vi "Version.vi"(8 "error in (no error)":errorcluster, 11 "S4GUI in":refnum<class "S4GUI.lvclass">) -> (0 "error out":errorcluster, 3 "S4GUI out":refnum<class "S4GUI.lvclass">)   [LabVIEW 2018, in "S4GUI.lvclass"]
uses:
  S4GUI.lvclass
  S4GUI.lvclass/S4GUI.ctl
  SyncBox/Sync Box.lvclass
  Acquisition/Acquisition.lvclass
  Instrument/Instrument.lvclass
  TCS/TCS.lvclass
  TelFocus/TelFocus.lvclass
  WeatherStation/WeatherStation.lvclass
  GSserver/GSserver.lvclass
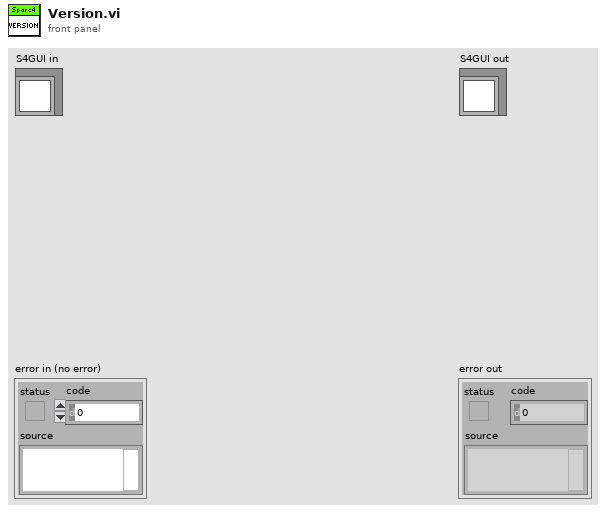
[diagram p1: front panel]
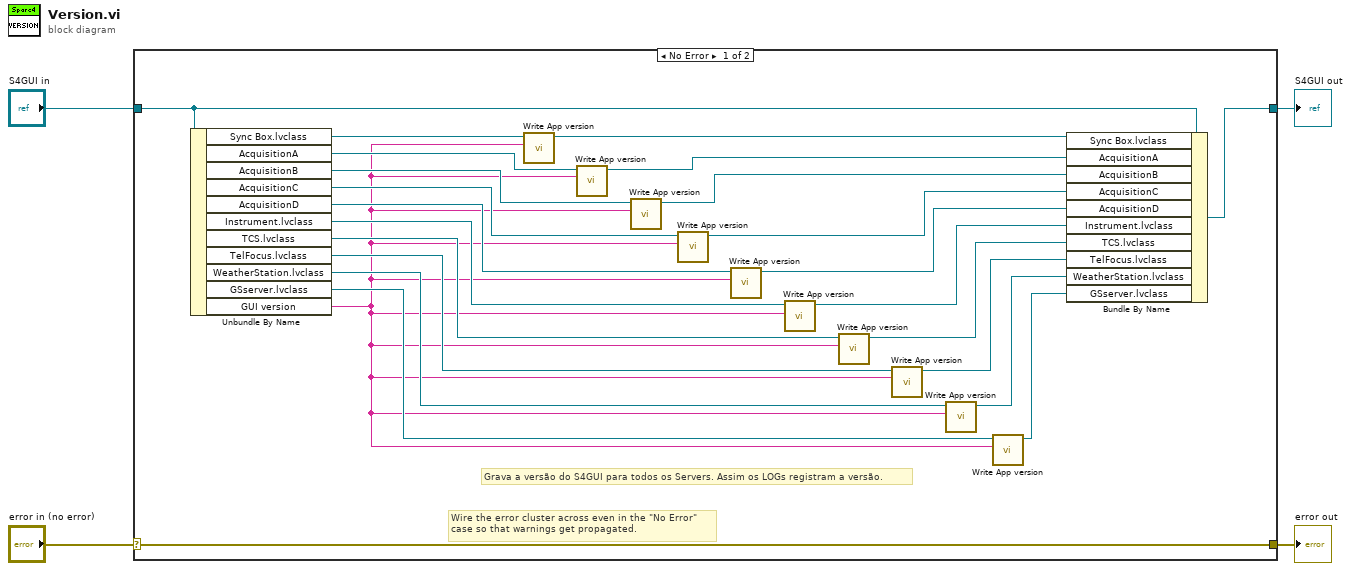
[diagram p0: block diagram]
diagram:
  n1 = case shown="No Error" "error in (no error)" {
    selector: "error in (no error)" -> [w28 w30]
    tunnel: [w28 w30] -> w3
    tunnel: [w15 w29] -> w1
    tunnel: "S4GUI in" -> [w16 w29]
    frame No Error {
      # "Grava a versão do S4GUI para todos os Servers. Assim os LOGs registram a versão."
      # "Wire the error cluster across even in the \"No Error\"\ncase so that warnings get propagated."
      n2 = Unbundle By Name(w16) -> ("Sync Box.lvclass"=w27:refnum<class "Sync Box.lvclass">, "AcquisitionA"=w26:refnum<class "Acquisition.lvclass">, "AcquisitionB"=w25:refnum<class "Acquisition.lvclass">, "AcquisitionC"=w24:refnum<class "Acquisition.lvclass">, "AcquisitionD"=w23:refnum<class "Acquisition.lvclass">, "Instrument.lvclass"=w22:refnum<class "Instrument.lvclass">, "TCS.lvclass"=w21:refnum<class "TCS.lvclass">, "TelFocus.lvclass"=w20:refnum<class "TelFocus.lvclass">, "WeatherStation.lvclass"=w19:refnum<class "WeatherStation.lvclass">, "GSserver.lvclass"=w18:refnum<class "GSserver.lvclass">, "GUI version"=w17:string)
      n3 = call-dynamic "Write App version.vi"("App version"=w17, "Server in"=w27) -> ("Server out"=w9:refnum<class "Sync Box.lvclass">)  [unwired: 8 in, 1 out]
      n4 = call-dynamic "Write App version.vi"("App version"=w17, "Server in"=w26) -> ("Server out"=w8:refnum<class "Acquisition.lvclass">)  [unwired: 8 in, 1 out]
      n5 = call-dynamic "Write App version.vi"("App version"=w17, "Server in"=w25) -> ("Server out"=w7:refnum<class "Acquisition.lvclass">)  [unwired: 8 in, 1 out]
      n6 = call-dynamic "Write App version.vi"("App version"=w17, "Server in"=w24) -> ("Server out"=w6:refnum<class "Acquisition.lvclass">)  [unwired: 8 in, 1 out]
      n7 = call-dynamic "Write App version.vi"("App version"=w17, "Server in"=w23) -> ("Server out"=w5:refnum<class "Acquisition.lvclass">)  [unwired: 8 in, 1 out]
      n8 = call-dynamic "Write App version.vi"("App version"=w17, "Server in"=w22) -> ("Server out"=w10:refnum<class "Instrument.lvclass">)  [unwired: 8 in, 1 out]
      n9 = call-dynamic "Write App version.vi"("App version"=w17, "Server in"=w21) -> ("Server out"=w11:refnum<class "TCS.lvclass">)  [unwired: 8 in, 1 out]
      n10 = call-dynamic "Write App version.vi"("App version"=w17, "Server in"=w20) -> ("Server out"=w12:refnum<class "TelFocus.lvclass">)  [unwired: 8 in, 1 out]
      n11 = call-dynamic "Write App version.vi"("App version"=w17, "Server in"=w19) -> ("Server out"=w13:refnum<class "WeatherStation.lvclass">)  [unwired: 8 in, 1 out]
      n12 = call-dynamic "Write App version.vi"("App version"=w17, "Server in"=w18) -> ("Server out"=w14:refnum<class "GSserver.lvclass">)  [unwired: 8 in, 1 out]
      n13 = Bundle By Name(cluster=w16, "Sync Box.lvclass"=w9, "AcquisitionA"=w8, "AcquisitionB"=w7, "AcquisitionC"=w6, "AcquisitionD"=w5, "Instrument.lvclass"=w10, "TCS.lvclass"=w11, "TelFocus.lvclass"=w12, "WeatherStation.lvclass"=w13, "GSserver.lvclass"=w14) -> (w15:refnum<class "S4GUI.lvclass">)
    }
    frame Error {
    }
  }
  "error out" <- w3
  "S4GUI out" <- w1
